vi "Text_To_Array (SubVI).vi"(8 "error in (no error)":errorcluster, 11 "Path":path) -> (0 "error out":errorcluster, 2 "text":string, 3 "Array":string[](array[string]))   [LabVIEW 2013]
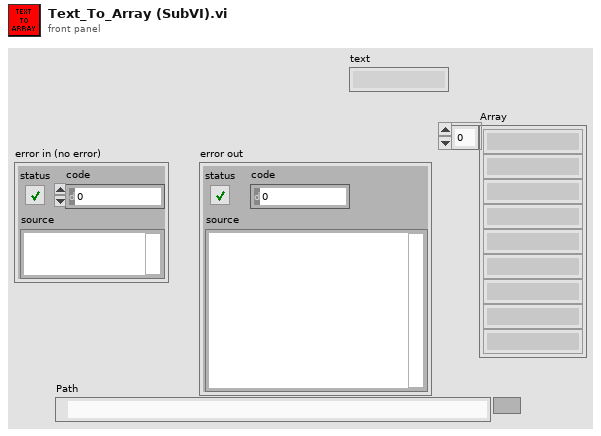
[diagram p1: front panel]
types:
  T1 = enum16{"open", "replace", "create", "open or create", "replace or create", "replace or create with confirmation"}
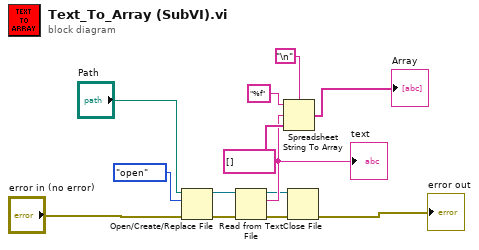
[diagram p0: block diagram]
diagram:
  n1 = Open/Create/Replace File(file path (use dialog)="Path", error in="error in (no error)", operation (0:open)=T1."open") -> (refnum out=w2:refnum<file>, error out=w3:errorcluster)  [unwired: 3 in, 1 out]
  n2 = Read from Text File(file (use dialog)=w2, error in=w3) -> (refnum out=w6:refnum<file>, text=w9:string, error out=w5:errorcluster)  [unwired: 2 in, 1 out]
  "text" <- w9
  n3 = Spreadsheet String To Array(delimiter (Tab)="\n", format string="%f", spreadsheet string=w9, array type (2D Dbl)=string[] []) -> (array=→"Array":string[])
  n4 = Close File(refnum=w6, error in=w5) -> (error out=→"error out":errorcluster)  [unwired: 1 out]
